vi "Untitled 2.vi"() -> ()   [LabVIEW 2019]
panel:
  out "error out":errorcluster
  out "Write OK":bool
  in  "UMBRAL TH0 (HLTH)":u8 format="%0x"
  out "Write OK 2":bool
  out "HANDLE":u32
  out "Error (\"1\" Error)":bool
  out "Todos":T1(array[cluster])=[{"Device Index"=0, "FT_FLAGS_OPENED"=TRUE, "FT_FLAGS_HISPEED"=TRUE, "Type"=6, "VID"=1027, "PID"=24592, "LocID"=1131585, "Serial Number"="CTAV2022A", "Description"="MI CTA TEST A", "FT_Handle"=433820616}, {"Device Index"=1, "FT_FLAGS_OPENED"=TRUE, "FT_FLAGS_HISPEED"=TRUE, "Type"=6, "VID"=1027, "PID"=24592, "LocID"=1131586, "Serial Number"="CTAV2022B", "Description"="MI CTA TEST B", "FT_Handle"=433822896}]
  out "Array CTA":T1(array[cluster])=[{"Device Index"=0, "FT_FLAGS_OPENED"=TRUE, "FT_FLAGS_HISPEED"=TRUE, "Type"=6, "VID"=1027, "PID"=24592, "LocID"=1131585, "Serial Number"="CTAV2022A", "Description"="MI CTA TEST A", "FT_Handle"=433820616}]
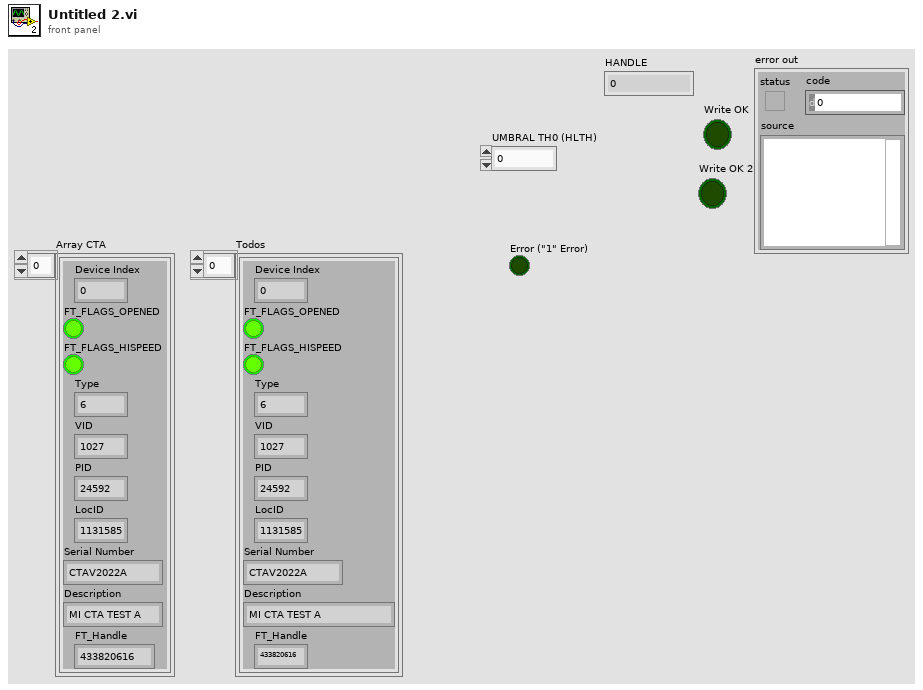
[diagram p1: front panel]
types:
  T1 = cluster{"Device Index":u32, "FT_FLAGS_OPENED":bool, "FT_FLAGS_HISPEED":bool, "Type":u32, "VID":u32, "PID":u32, "LocID":i32, "Serial Number":string, "Description":string, "FT_Handle":u32}[]
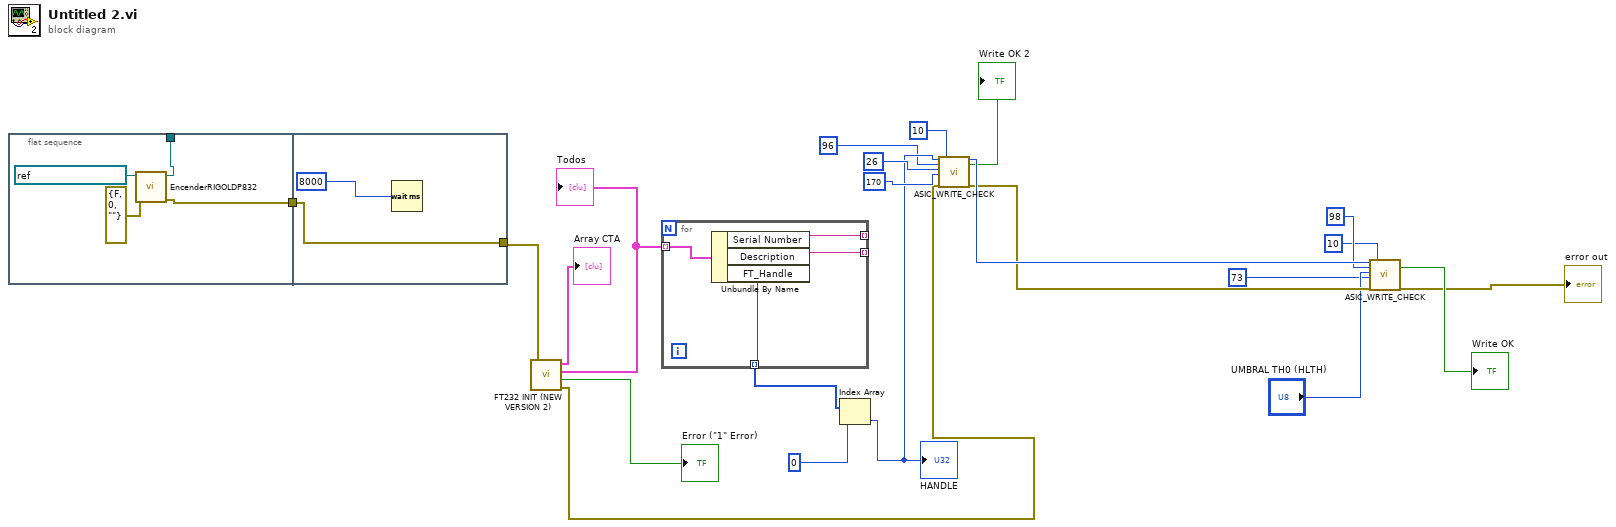
[diagram p0: block diagram]
diagram:
  n1 = flat-sequence {
    tunnel: [w25] -> _
    tunnel: [w24] -> w17
    tunnel: w17 -> [w27]
    tunnel: [w27] -> w16
    frame #0 {
      n2 = call "EncenderRIGOLDP832.vi"("error in (no error)"=errorcluster {"status"=FALSE, "code"=0, "source"=""}, "VISA IN"=refnum<visa-resource-name> "FA_Rigol_DP832") -> ("error out"=w24:errorcluster, "VISA resource name out"=w25:refnum<visa-resource-name>)  [unwired: 8 in]
    }
    frame #1 {
      n3 = Wait (ms)(milliseconds to wait=u32 8000) -> ()  [unwired: 1 out]
    }
  }
  n4 = call "FT232 INIT (NEW VERSION 2).vi"("error in (no error)"=w16) -> ("error out"=w3:errorcluster, "Error (\"1\" Error)"=→"Error (\"1\" Error)":bool, "Todos"=w21:T1, "Array CTA"=→"Array CTA":T1)  [unwired: 7 in]
  "Todos" <- w21
  n5 = for {
    tunnel: w21 -> [w32] mode=indexing
    tunnel: [w31] -> _ mode=indexing
    tunnel: [w30] -> _ mode=indexing
    tunnel: [w29] -> w22 mode=indexing
    n6 = Unbundle By Name(w32) -> ("Serial Number"=w31:string, "Description"=w30:string, "FT_Handle"=w29:u32)
  }
  n7 = Index Array(array=w22, index=0) -> (element=w2:u32)
  "HANDLE" <- w2
  n8 = call "ASIC_WRITE_CHECK.vi"("ftHandle_in"=w2, "Direccion Registro Asic"=u8 96, "Byte Alto"=u8 26, "Byte Bajo"=u8 170, "error in"=w3, "Espera acceso USB 2"=u32 10) -> ("ftHandle_out"=w13:u32, "Write OK"=→"Write OK 2":bool, "error out"=w11:errorcluster)  [unwired: 11 in]
  n9 = call "ASIC_WRITE_CHECK.vi"("ftHandle_in"=w13, "Direccion Registro Asic"=u8 98, "Byte Alto"="UMBRAL TH0 (HLTH)", "Byte Bajo"=u8 73, "error in"=w11, "Espera acceso USB 2"=u32 10) -> ("Write OK"=→"Write OK":bool, "error out"=→"error out":errorcluster)  [unwired: 11 in, 1 out]
